vi "Save3.vi"(1 "要保存的文件名（输入）":string="AI2.csv", 2 "数组中的数据（输入）":dbl[](array[numeric])) -> (0 "文件保存路径（输出）":path)   [LabVIEW 2018]
uses:
  <vilib>/Utility/error.llb/DialogType.ctl
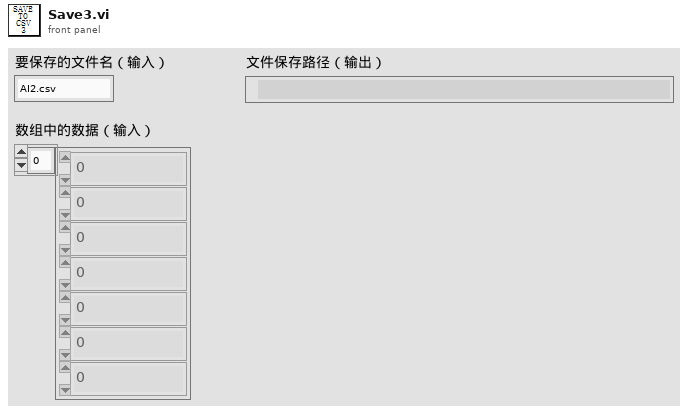
[diagram p1: front panel]
types:
  T1 = typedef "DialogType.ctl" = u16
  T2 = enum16{"open", "replace", "create", "open or create", "replace or create", "replace or create with confirmation"}
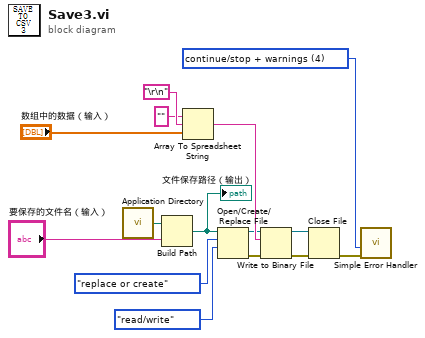
[diagram p0: block diagram]
diagram:
  w9 = T1 4 items=["no dialog", "OK message", "continue or stop message", "OK message + warnings", "continue/stop + warnings"] ("type of dialog (OK msg:1)")
  n1 = call <vilib>:"Application Directory.vi"() -> ("Application Directory"=w1:path)
  n2 = Build Path(base path=w1, name or relative path="要保存的文件名（输入）") -> (appended path=w2:path)
  "文件保存路径（输出）" <- w2
  n3 = Array To Spreadsheet String(delimiter (Tab)="\r\n", array="数组中的数据（输入）", 3:"" ("format string")) -> (spreadsheet string=w15:string)
  n4 = Open/Create/Replace File(file path (use dialog)=w2, operation (0:open)=T2."replace or create", access (0:read/write)=enum16{"read/write", "read-only", "write-only"}."read/write") -> (refnum out=w4:refnum<file>, error out=w5:errorcluster)  [unwired: 3 in, 1 out]
  n5 = Write to Binary File(file (use dialog)=w4, data=w15, error in=w5) -> (refnum out=w6:refnum<file>, error out=w7:errorcluster)  [unwired: 3 in, 1 out]
  n6 = Close File(refnum=w6, error in=w7) -> (error out=w8:errorcluster)  [unwired: 1 out]
  n7 = call <vilib>:"Simple Error Handler.vi"("type of dialog (OK msg:1)"=w9, "error in (no error)"=w8) -> ()  [unwired: 3 in, 5 out]
